vi "DoubleToUShort.vi"(1 "Value":dbl, 2 "Max":dbl, 3 "Min":dbl) -> (0 "scaled Integer":u16)   [LabVIEW 2009]
panel:
  out "Bias":dbl
  out "ScalingFactor":dbl
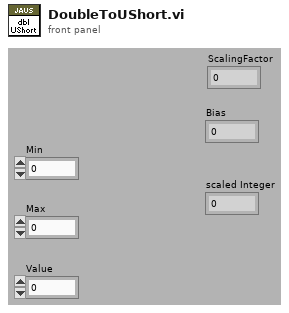
[diagram p1: front panel]
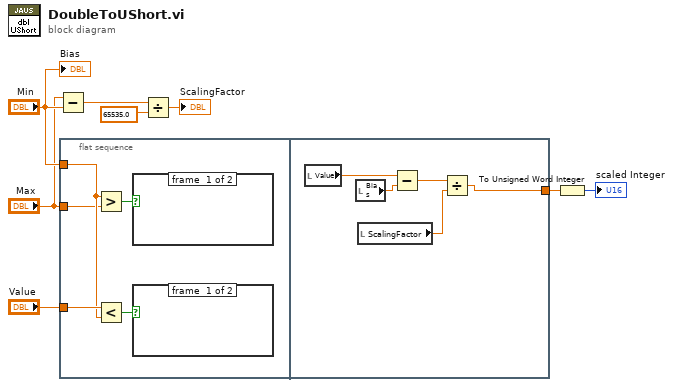
[diagram p0: block diagram]
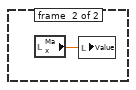
[diagram p2: hidden frame]
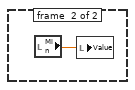
[diagram p3: hidden frame]
diagram:
  n1 = Subtract(x="Max", y="Min") -> (x-y=w8:dbl)
  n2 = flat-sequence {
    tunnel: "Value" -> [w13]
    tunnel: "Min" -> [w11]
    tunnel: "Max" -> [w10]
    tunnel: [w16] -> w2
    frame #0 {
      n3 = Greater?(x=w11, y=w10) -> (0:w9:bool)
      n4 = Less?(x=w13, y=w11) -> (x < y?=w12:bool)
      n5 = case shown="True" w9 {
        frame #0 {
        }
        frame #1 {
          n6 = local read "Max"() -> (w14:dbl)
          n7 = local write "Value"(w14) -> ()
        }
      }
      n8 = case shown="True" w12 {
        frame #0 {
        }
        frame #1 {
          n9 = local read "Min"() -> (w15:dbl)
          n10 = local write "Value"(w15) -> ()
        }
      }
    }
    frame #1 {
      n11 = local read "Value"() -> (w20:dbl)
      n12 = local read "Bias"() -> (w19:dbl)
      n13 = local read "ScalingFactor"() -> (w18:dbl)
      n14 = Subtract(x=w20, y=w19) -> (x-y=w17:dbl)
      n15 = Divide(x=w17, y=w18) -> (x/y=w16:dbl)
    }
  }
  n16 = Divide(x=w8, y=65535.0) -> (x/y=→"ScalingFactor":dbl)
  n17 = To Unsigned Word Integer(number=w2) -> (unsigned 16bit integer=→"scaled Integer":u16)
  "Bias" <- "Min"
